vi "Initialize From Path.vi"(7 "Path":path, 8 "error in (no error)":errorcluster, 9 "Build Configurations":string[](array[string]), 10 "Preceding Items":refnum<class "Item.lvclass">[](array[class]), 11 "VIPM Item in":refnum<class "VIPM Item.lvclass">) -> (0 "error out":errorcluster, 3 "Item out":refnum<class "Item.lvclass">)   [LabVIEW 2019, in "VIPM.lvlib" / "VIPM Item.lvclass"]
uses:
  VIPM Item.lvclass
  libs/Solution.lvlibp/Solution/Item/Item.lvclass
  C:/Users/pasca/source/repos/mgi-solution-explorer-extensions/libs/Solution.lvlibp/Solution/Item/Item.lvclass
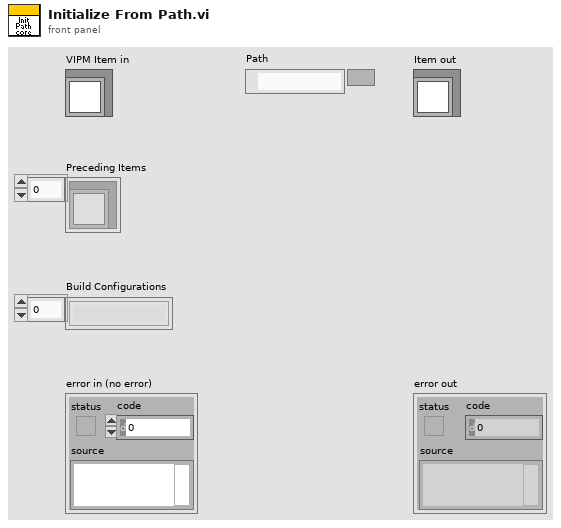
[diagram p1: front panel]
types:
  T1 = typedef "VIPM.lvlib/VIPM Item.lvclass/File Type.ctl" = enum16{"Unsupported", "VIPB", "VIPC"}
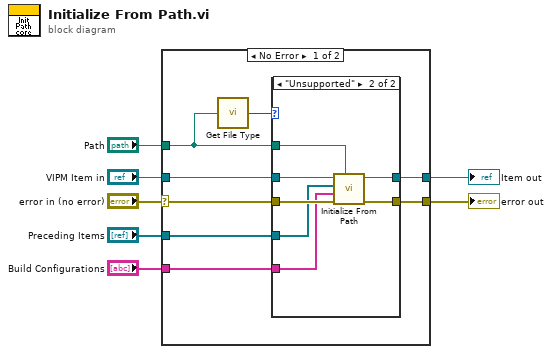
[diagram p0: block diagram]
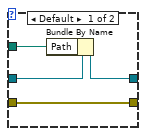
[diagram p2: hidden frame]
diagram:
  n1 = case shown="No Error" "error in (no error)" {
    selector: "error in (no error)" -> [w13 w27]
    tunnel: [w15 w27] -> w7
    tunnel: [w14 _] -> w6
    tunnel: "Path" -> [w8 _]
    tunnel: "Build Configurations" -> [w12 _]
    tunnel: "Preceding Items" -> [w11 _]
    tunnel: "VIPM Item in" -> [w10 _]
    frame No Error {
      n2 = call "Get File Type.vi"("Path"=w8) -> ("File Type"=w9:T1)  [unwired: 1 in]
      n3 = case shown="\"Unsupported\"" w9 {
        tunnel: [w16 w26] -> w15
        tunnel: [w18 w25] -> w14
        tunnel: w8 -> [w17 w24]
        tunnel: w13 -> [w16 w23]
        tunnel: w12 -> [_ w22]
        tunnel: w11 -> [_ w21]
        tunnel: w10 -> [w19 w20]
        frame Default {
          n4 = Bundle By Name(cluster=w19, "Path"=w17) -> (w18:refnum<class "VIPM Item.lvclass">)
        }
        frame "Unsupported" {
          n5 = call-parent "Initialize From Path.vi"("Path"=w24, "error in (no error)"=w23, "Build Configurations"=w22, "Preceding Items"=w21, "Item in"=w20) -> ("error out"=w26:errorcluster, "Item out"=w25:refnum<class "Item.lvclass">)  [unwired: 5 in]
        }
      }
    }
    frame Error {
    }
  }
  "error out" <- w7
  "Item out" <- w6
